vi "Q8381 X_Axis E Off.vi"(1 "Graph Data":T1 {"Y Axis Data" format="%.5e"; "X Axis Data" format="%.5e"}) -> (0 "Out Data":T1 {"Y Axis Data" format="%.5e"; "X Axis Data" format="%.5f"})   [LabVIEW 2017]
doc: "Cut off \"E\" and after to show unit-free X-axis value. (Cut off is done by multiplying one million to X Axis Data)\n Input: Cluster of 2 arrays:\n X Axis Data: DBL\n Y Axis Data: DBL\n Output:Cluster of 2 arrays:\n X Axis Data: DBL\n Y Axis Data: DBL"
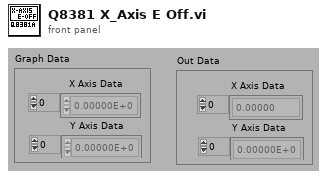
[diagram p1: front panel]
types:
  T1 = cluster{"X Axis Data":dbl[], "Y Axis Data":dbl[]}
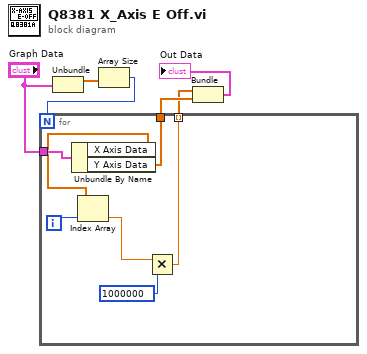
[diagram p0: block diagram]
diagram:
  n1 = Unbundle("Graph Data") -> ("X Axis Data"=w2:dbl[])  [unwired: 1 out]
  n2 = Array Size(array=w2) -> (size(s)=w1:i32)
  n3 = for {
    N: w1 -> [_]
    tunnel: "Graph Data" -> [w10]
    tunnel: [w9] -> w5
    tunnel: [w8] -> w4 mode=indexing
    i -> [w13]
    n4 = Unbundle By Name(w10) -> ("X Axis Data"=w7:dbl[], "Y Axis Data"=w9:dbl[])
    n5 = Index Array(array=w7, index=w13) -> (element=w12:dbl)
    n6 = Multiply(x=w12, y=1000000) -> (x*y=w8:dbl)
  }
  n7 = Bundle(w4, "Y Axis Data"=w5) -> (→"Out Data":cluster{dbl[], "Y Axis Data":dbl[]})  [unwired: 1 in]
